vi "UHR-Fleezers Control (host) - Lorentz v3.vi"() -> ()   [LabVIEW 2014] (continued)
            n2217 = property on="APD 2"() -> ("Displayed Image Position"=w3357)  [unwired: 2 in, 2 out]
            n2218 = property on="APD 1"() -> ("Displayed Image Position"=w3386)  [unwired: 2 in, 2 out]
            n2219 = property on="Detection Laser X"() -> ("Displayed Image Position"=w3383)  [unwired: 2 in, 2 out]
            n2220 = property on="Detection Laser Y"() -> ("Displayed Image Position"=w3382)  [unwired: 2 in, 2 out]
            n2221 = Unbundle By Name(w3356) -> ("Width"=w3353, "Height"=w3352)
            n2222 = Unbundle By Name(w3357) -> ("Left"=w3355, "Top"=w3354)
            n2223 = Unbundle By Name(w3384) -> ("Width"=w3378, "Height"=w3377)
            n2224 = Unbundle By Name(w3385) -> ("Width"=w3374, "Height"=w3373)
            n2225 = Unbundle By Name(w3381) -> ("Width"=w3370, "Height"=w3369)
            n2226 = Unbundle By Name(w3386) -> ("Left"=w3380, "Top"=w3379)
            n2227 = Unbundle By Name(w3383) -> ("Left"=w3376, "Top"=w3375)
            n2228 = Unbundle By Name(w3382) -> ("Left"=w3372, "Top"=w3371)
            n2229 = Bundle("Left"=w3355, "Top"=w3354, "Width"=w3353, "Height"=w3352) -> (w3351:T49)  [unwired: 1 in]
            n2230 = Bundle("Left"=w3380, "Top"=w3379, "Width"=w3378, "Height"=w3377) -> (w3368:T49)  [unwired: 1 in]
            n2231 = Bundle("Left"=w3376, "Top"=w3375, "Width"=w3374, "Height"=w3373) -> (w3367:T49)  [unwired: 1 in]
            n2232 = Bundle("Left"=w3372, "Top"=w3371, "Width"=w3370, "Height"=w3369) -> (w3366:T49)  [unwired: 1 in]
            n2233 = Build Cluster Array(w3351, w3368, w3367, w3366) -> (w3365:T50)
            n2234 = for {
              tunnel: w3387 -> [w3398]
              tunnel: w3365 -> [w3399] mode=indexing
              shift-right: [w3396] -> w3363
              shift-left: TRUE -> [w3397]
              shift-right: [w3395] -> w3361
              shift-left: _ -> [w3391]
              shift-right: [w3394] -> w3360
              shift-left: _ -> [w3390]
              shift-right: [w3393] -> w3359
              shift-left: _ -> [w3389]
              shift-right: [w3392] -> w3358
              shift-left: _ -> [w3388]
              n2235 = case shown="True" w3397 {
                selector: w3397 -> [w3404 _]
                tunnel: w3399 -> [_ w3413]
                tunnel: w3398 -> [_ w3411]
                tunnel: [w3404 w3409] -> w3396
                tunnel: [w3403 w3408] -> w3395
                tunnel: [w3402 w3407] -> w3394
                tunnel: [w3401 w3406] -> w3393
                tunnel: [w3400 w3405] -> w3392
                tunnel: w3391 -> [w3403 _]
                tunnel: w3390 -> [w3402 _]
                tunnel: w3389 -> [w3401 _]
                tunnel: w3388 -> [w3400 _]
                frame False {
                }
                frame True {
                  n2236 = Unbundle(w3413) -> (w3412:T49)
                  n2237 = call "isclickinwindow.vi"("Image Param"=w3412, "Point32"=w3411) -> ("4 Y"=w3405:i32, "3 Height"=w3406:i32, "2 X"=w3407:i32, "1 Width"=w3408:i32, "In image?"=w3410:bool)  [unwired: 1 in]
                  n2238 = Not(x=w3410) -> (.not. x?=w3409:bool)
                }
              }
            }
            n2239 = Not(x=w3363) -> (.not. x?=w3362:bool)
            n2240 = case shown="True" w3362 {
              tunnel: w3360 -> [_ w3427]
              tunnel: w3358 -> [_ w3426]
              tunnel: w3361 -> [_ w3425]
              tunnel: w3359 -> [_ w3424]
              frame False {
              }
              frame True {
                w3414 = FALSE ("Get Point")
                n2241 = local read "Scan lines (y)"() -> (w3429:u64)
                n2242 = disable-structure shown="Disabled" {
                  frame Disabled {
                  }
                  frame Enabled {
                  }
                }
                n2243 = local read "Actual MCL Inc (V)"() -> (w3423:dbl)
                n2244 = local read "Scan steps (MCL)"() -> (w3428:u64)
                n2245 = Divide "Y Pix/step"(x=w3424, y=w3429) -> (x/y=w3436:dbl)
                n2246 = Divide "Y V/pix"(x=w3423, y=w3436) -> (x/y=w3435:dbl)
                n2247 = Divide "Y half step offset"(x=w3423, y=2.0) -> (x/y=w3437:dbl)
                n2248 = Divide "X pix/step"(x=w3425, y=w3428) -> (x/y=w3434:dbl)
                n2249 = Negate(x=w3437) -> (-x=w3438:dbl)
                n2250 = local read "Initial Y"() -> (w3444:dbl)
                n2251 = Multiply(x=w3426, y=w3435) -> (x*y=w3445:dbl)
                n2252 = Divide "X half step offset"(x=w3423, y=2.0) -> (x/y=w3431:dbl)
                n2253 = Divide "X V/pix"(x=w3423, y=w3434) -> (x/y=w3433:dbl)
                n2254 = Multiply(x=w3423, y=w3428) -> (x*y=w3440:dbl)
                n2255 = Compound Arithmetic op=ADD(w3438, w3445, w3444) -> (w3415:dbl)
                "Pointer Y (V)" <- w3415
                n2256 = Multiply(x=w3433, y=w3427) -> (x*y=w3442:dbl)
                n2257 = Negate(x=w3431) -> (-x=w3430:dbl)
                n2258 = local read "Initial X"() -> (w3443:dbl)
                n2259 = Negate(x=w3442) -> (-x=w3441:dbl)
                n2260 = Compound Arithmetic op=ADD(w3430, w3440, w3443, w3441) -> (w3416:dbl)
                "Pointer X (V)" <- w3416
                n2261 = case shown="True" "Set High F Confocal Spot (X-Y)" {
                  tunnel: w3416 -> [_ w3446]
                  tunnel: w3415 -> [_ w3447]
                  frame False {
                  }
                  frame True {
                    "Confocal Y 2 (V)" <- w3447
                    "Confocal X 2 (V)" <- w3446
                  }
                }
                n2262 = Or(x="Set X Only", y="Set Confocal Spot (X-Y)") -> (x .or. y?=w3419:bool)
                n2263 = Or(x="Set Confocal Spot (X-Y)", y="Set Y Only") -> (x .or. y?=w3418:bool)
                n2264 = case shown="True" w3419 {
                  tunnel: w3416 -> [_ w3448]
                  frame False {
                  }
                  frame True {
                    n2265 = property on="AO2" class="Slide (strict)"("Val(Sgnl)"=w3448) -> ()  [unwired: 2 in, 2 out]
                    "Confocal X 1 (V)" <- w3448
                  }
                }
                n2266 = case shown="True" w3418 {
                  tunnel: w3415 -> [_ w3449]
                  frame False {
                  }
                  frame True {
                    n2267 = property on="AO1" class="Slide (strict)"("Val(Sgnl)"=w3449) -> ()  [unwired: 2 in, 2 out]
                    "Confocal Y 1 (V)" <- w3449
                  }
                }
                n2268 = local write "Set High F Confocal Spot (X-Y)"(w3414) -> ()
                n2269 = local write "Set Confocal Spot (X-Y)"(w3414) -> ()
                n2270 = local write "Set X Only"(w3414) -> ()
                n2271 = local write "Set Y Only"(w3414) -> ()
              }
            }
          }
          frame 3 {
            n2272 = local read "BD 2 Frequency 1 (MHz)"() -> (w3451:dbl)
            n2273 = local read "BD 1 Frequency 1 (MHz)"() -> (w3452:dbl)
            n2274 = local write "Manipulating Trap"(TRUE ("Manipulating Trap")) -> ()
            n2275 = local write "Coords"(T12 {"Horizontal"=0, "Vertical"=0} ("Coords")) -> ()
            n2276 = while {
              tunnel: w3456 -> [w3461]
              tunnel: w3454 -> [w3460]
              tunnel: w3452 -> [w3459]
              tunnel: w3451 -> [w3458]
              tunnel: w3450 -> [w3457]
              stop <- w3462 stop-if-true
              n2277 = event shown="[0] \"Pane\": Mouse Move" {
                selector: _ -> [_ _]
                dyn-events: _ -> [_ _]
                timeout: _ -> [_ _]
                tunnel: ["Force Manip Abort" w3526] -> w3462
                tunnel: w3461 -> [w3469 _]
                tunnel: w3460 -> [w3467 _]
                tunnel: w3459 -> [w3466 _]
                tunnel: w3458 -> [w3465 _]
                tunnel: w3457 -> [w3463 _]
                event Mouse Move {
                  n2278 = event-data() -> ("Time"=w3470:u32, "Coords"=w3471:T12)  [unwired: 3 out]
                  n2279 = Less?(x=w3470, y=w3469) -> (x < y?=w3468:bool)
                  n2280 = case "Makes sure old motion events prior to mouse click aren't used" shown="False" w3468 {
                    tunnel: w3471 -> [w3513 _]
                    tunnel: w3467 -> [w3514 _]
                    tunnel: w3466 -> [w3488 _]
                    tunnel: w3465 -> [w3487 _]
                    tunnel: w3463 -> [w3472 _]
                    frame False {
                      n2281 = Subtract(x=w3513, y=w3514) -> (x-y=w3512:T12)
                      "Coords" <- w3512
                      n2282 = local read "Y RF Frequency Limits (MHz)"() -> (w3473:T24)
                      n2283 = To Double Precision Float(number=w3512) -> (double precision float=w3511:cluster{"Horizontal":dbl, "Vertical":dbl})
                      n2284 = Multiply(x=cluster{"Horizontal":dbl, "Vertical":dbl} {"Horizontal"=-1.0, "Vertical"=1.0}, y="Manipulation Scaling") -> (x*y=w3507:cluster{"Horizontal":dbl, "Vertical":dbl})
                      n2285 = local read "X RF Frequency Limits (MHz)"() -> (w3474:T24)
                      n2286 = Multiply(x=w3511, y=w3507) -> (x*y=w3509:cluster{"Horizontal":dbl, "Vertical":dbl})
                      n2287 = Unbundle By Name(w3509) -> ("Horizontal"=w3504:dbl, "Vertical"=w3508:dbl)
                      n2288 = Unbundle By Name(w3473) -> ("Maximum"=w3476:dbl, "Minimum"=w3475:dbl)
                      n2289 = Boolean To (0,1)(Boolean="Manip. X?") -> (0, 1=w3502:i16)
                      n2290 = Boolean To (0,1)(Boolean="Manip. Y?") -> (0, 1=w3499:i16)
                      n2291 = local read "BD 1 Frequency 2 (MHz)"() -> (w3490:dbl)
                      n2292 = Multiply(x=w3508, y=w3499) -> (x*y=w3501:dbl)
                      n2293 = Multiply(x=w3502, y=w3504) -> (x*y=w3505:dbl)
                      n2294 = local read "BD 2 Frequency 2 (MHz)"() -> (w3489:dbl)
                      n2295 = Unbundle By Name(w3474) -> ("Maximum"=w3478:dbl, "Minimum"=w3477:dbl)
                      n2296 = Add(x=w3487, y=w3501) -> (x+y=w3480:dbl)
                      n2297 = Add(x=w3488, y=w3505) -> (x+y=w3482:dbl)
                      n2298 = In Range and Coerce(upper limit=w3478, x=w3482, lower limit=w3477) -> (coerced(x)=w3481:dbl)  [unwired: 1 out]
                      n2299 = In Range and Coerce(upper limit=w3476, x=w3480, lower limit=w3475) -> (coerced(x)=w3479:dbl)  [unwired: 1 out]
                      n2300 = Subtract(x=w3481, y=w3490) -> (x-y=w3498:dbl)
                      n2301 = Subtract(x=w3479, y=w3489) -> (x-y=w3497:dbl)
                      n2302 = Square(x=w3498) -> (x^2=w3496:dbl)
                      n2303 = Square(x=w3497) -> (x^2=w3495:dbl)
                      n2304 = Add(x=w3496, y=w3495) -> (x+y=w3494:dbl)
                      n2305 = Square Root(x=w3494) -> (sqrt(x)=w3491:dbl)
                      n2306 = In Range and Coerce(upper limit="Limit Max (MHz)", x=w3491, lower limit="Limit Min (MHz)") -> (In Range?=w3484:bool)  [unwired: 1 out]
                      n2307 = Not(x="Limits Enable") -> (.not. x?=w3483:bool)
                      n2308 = Or(x=w3484, y=w3483) -> (x .or. y?=w3485:bool)
                      n2309 = case shown="True" w3485 {
                        tunnel: w3491 -> [_ w3516]
                        tunnel: w3481 -> [_ w3523]
                        tunnel: w3490 -> [_ w3522]
                        tunnel: w3479 -> [_ w3521]
                        tunnel: w3489 -> [_ w3520]
                        tunnel: w3474 -> [_ w3518]
                        tunnel: w3473 -> [_ w3517]
                        tunnel: w3472 -> [_ w3515]
                        frame False {
                        }
                        frame True {
                          n2310 = local read "BD 1 Frequency 3 (MHz)"() -> (w3524:dbl)
                          n2311 = local read "BD 2 Frequency 3 (MHz)"() -> (w3519:dbl)
                          n2312 = local write "Trap Delta (MHz)"(w3516) -> ()
                          n2313 = call "set RF board frequency - interlace.vi"("Board 2 Frequency Limits"=w3517, "Board 1 Frequency Limits"=w3518, "FPGA VI Reference In"=w3515, "Board 2 Frequency 3 (MHz)"=w3519, "Board 1 Frequency 3 (MHz)"=w3524, "Board 2 Frequency 2 (MHz)"=w3520, "Board 2 Frequency 1 (MHz)"=w3521, "Board 1 Frequency 2 (MHz)"=w3522, "Board 1 Frequency 1  (MHz)"=w3523) -> ()  [unwired: 1 in, 2 out]
                          n2314 = local write "BD 2 Frequency 1 (MHz)"(w3521) -> ()
                          n2315 = local write "BD 1 Frequency 1 (MHz)"(w3523) -> ()
                        }
                      }
                    }
                    frame True {
                    }
                  }
                }
                event Mouse Up {
                  n2316 = event-data() -> ("Button"=w3525:u16)  [unwired: 8 out]
                  n2317 = case shown="3" w3525 {
                    tunnel: [FALSE TRUE] -> w3526
                    frame 0, Default {
                    }
                    frame 3 {
                      n2318 = local read "Trap Delta (MHz)"() -> (w3528:dbl)
                      n2319 = property on="Initial delta (MHz)" class="DigNum (strict)"("Val(Sgnl)"=w3528) -> ()  [unwired: 2 in, 2 out]
                      n2320 = local write "Manipulating Trap"(FALSE ("Manipulating Trap")) -> ()
                    }
                  }
                }
              }
            }
          }
        }
      }
      event Timeout {
        n2321 = event-data() -> ()  [unwired: 4 out]
      }
      event "Stop All": Mouse Down {
        n2322 = event-data() -> ()  [unwired: 9 out]
      }
      event Mouse Move {
        n2323 = event-data() -> ()  [unwired: 6 out]
      }
    }
    n2324 = node-c288() -> ()  [unwired: 2 out]
  }
  n2325 = node-c288(3 ("Processor")) -> (w63:T37)  [unwired: 3 out]
  n2326 = node-c288(i64 1 ("Period"), 1 ("Processor")) -> (w71:T37)  [unwired: 2 in, 2 out]
  n2327 = timed-loop "Oscillate Trap/AOM (fishing, conjugate plane alignment)" {
    tunnel: [w3534] -> w68
    timing: w63 -> [_]
    timing-out: [_] -> w62
    tunnel: w24 -> [w3533]
    tunnel: w12 -> [w3532]
    stop <- w3534 stop-if-true
    n2328 = node-c288() -> ()  [unwired: 2 out]
    n2329 = event shown="[2] \"Start assembly line\": Value Change" {
      selector: _ -> [_ _ _ _]
      dyn-events: _ -> [_ _ _ _]
      timeout: _ -> [_ _ _ _]
      tunnel: [FALSE ("Stop All") _ _ w4207] -> w3534
      tunnel: w3533 -> [w3537 _ _ _]
      tunnel: w3532 -> [_ _ w4142 _]
      event "Oscillate Set 1", "Fish for Tether": Value Change {
        n2330 = event-data() -> ()  [unwired: 6 out]
        n2331 = local read "Oscillate Set 1"() -> (w3541:bool)
        n2332 = Or(x=w3541, y="Fish for Tether") -> (x .or. y?=w3539:bool)
        n2333 = case shown="True" w3539 {
          tunnel: "Fish for Tether" -> [_ w3544]
          tunnel: w3537 -> [_ w3542]
          frame False {
          }
          frame True {
            n2334 = case shown="True" w3544 {
              selector: w3544 -> [w3547 w3553]
              tunnel: [w3547 w3553] -> w3543
              frame False {
              }
              frame True {
                n2335 = local write "Scan axis 2"(TRUE) -> ()
                n2336 = local write "Tether"(FALSE ("Tether")) -> ()
                n2337 = local read "Flow ON during cal?"() -> (w3548:bool)
                n2338 = property on="Trap Delta (MHz)" class="DigNum (strict)"("Val(Sgnl)"="Furthest Delta (MHz)") -> ()  [unwired: 2 in, 2 out]
                n2339 = Or(x="Flow ON during \nfishing?", y=w3548) -> (x .or. y?=w3549:bool)
                n2340 = Wait (ms)(milliseconds to wait=u32 500) -> ()  [unwired: 1 out]
                n2341 = property on="Sample Channel\nFlow" class="Bool (strict)"("Val(Sgnl)"=w3549) -> ()  [unwired: 2 in, 2 out]
              }
            }
            n2342 = node-c288() -> (w3546:T37)  [unwired: 1 in, 3 out]
            n2343 = timed-loop "Oscillate AOD" {
              timing: w3546 -> [_]
              timing-out: [_] -> w3545
              tunnel: w3543 -> [w3557]
              tunnel: w3542 -> [w3556]
              i -> [w3565]
              stop <- w3563 stop-if-true
              n2344 = node-c288() -> (w3564:i64)  [unwired: 1 out]
              n2345 = flat-sequence {
                tunnel: w3565 -> [w3592]
                tunnel: w3564 -> [w3591]
                tunnel: w3557 -> [w3575]
                tunnel: [w3575] -> w3562
                tunnel: [w3574] -> w3561
                tunnel: [w3573] -> w3560
                tunnel: [w3570] -> w3558
                tunnel: w3556 -> [w3566]
                tunnel: w3562 -> [w3639]
                tunnel: w3561 -> [w3637]
                tunnel: w3560 -> [w3636]
                tunnel: [w3635] -> w3559
                tunnel: w3558 -> [w3634]
                tunnel: [w3711] -> w3563
                tunnel: w3559 -> [w3710]
                frame #0 {
                  # "w (rad/s)"
                  # "t (s)"
                  n2346 = Divide(x=w3591, y=i64 1000) -> (x/y=w3567:dbl)
                  n2347 = local read "BD 1 Frequency 2 (MHz)"() -> (w3569:dbl)
                  n2348 = Multiply(x="Osc. freq. (Hz)", y=6.283185307179586) -> (x*y=w3589:dbl)
                  n2349 = Multiply(x=w3567, y=w3592) -> (x*y=w3588:dbl)
                  n2350 = Multiply(x=w3589, y=w3588) -> (x*y=w3572:dbl)
                  n2351 = local read "BD 1 Frequency 1 (MHz)"() -> (w3577:dbl)
                  n2352 = case shown="True" w3575 {
                    tunnel: w3572 -> [w3598 w3617]
                    tunnel: w3577 -> [_ w3625]
                    tunnel: w3569 -> [_ w3626]
                    tunnel: [w3595 w3621] -> w3568
                    tunnel: [FALSE w3599] -> w3573
                    tunnel: [0.0 w3613] -> w3570
                    frame False {
                      n2353 = Sine(x=w3598) -> (sin(x)=w3596:dbl)
                      n2354 = Multiply(x=w3596, y="Osc. amp. (MHz)") -> (x*y=w3595:dbl)
                    }
                    frame True {
                      # "trap position goes from 0 to 1 (0 is when it is furthest away, 1 is when closest)\nso we want to test for tether only when farther away, or x < 1"
                      # "quit if taking too long"
                      # "oscillate the trap"
                      # "Test for tether"
                      n2355 = local read "Vec Mean of T1 T2"() -> (w3602:dbl[])
                      "Trigger Signal" <- w3602
                      n2356 = Cosine(x=w3617) -> (cos(x)=w3629:dbl)
                      n2357 = Subtract(x=w3626, y=w3625) -> (x-y=w3624:dbl)
                      n2358 = Decrement(x=w3629) -> (x-1=w3628:dbl)
                      n2359 = Subtract(x=w3624, y="Closest Delta (MHz)") -> (x-y=w3622:dbl)
                      n2360 = Divide(x=w3628, y=-2.0) -> (x/y=w3612:dbl)
                      n2361 = Greater?(x=w3602, y="Stop F (pN)") -> (0:w3619:bool[])
                      n2362 = Multiply(x=w3612, y=w3622) -> (x*y=w3621:dbl)
                      n2363 = Less?(x=w3612, y="Fish mask thresh") -> (x < y?=w3611:bool)
                      n2364 = Boolean To (0,1)(Boolean=w3611) -> (0, 1=w3609:i16)
                      n2365 = Multiply(x=w3609, y=w3602) -> (x*y=w3608:dbl[])
                      n2366 = Divide(x=w3617, y=6.283185307179586) -> (x/y=w3616:dbl)
                      n2367 = Round Toward +Infinity(x=w3616) -> (ceil(x): smallest int >= x=w3613:dbl)
                      "Attempts" <- w3613
                      n2368 = Greater?(x=w3608, y="Stop F (pN) (mask)") -> (0:w3606:bool[])
                      n2369 = Or Array Elements(Boolean array=w3619) -> (logical OR=w3604:bool)
                      n2370 = Or Array Elements(Boolean array=w3606) -> (logical OR=w3603:bool)
                      n2371 = Greater?(x=w3613, y="Attempt Limit") -> (0:w3615:bool)
                      n2372 = case shown="True" w3615 {
                        frame False {
                        }
                        frame True {
                          n2373 = local write "Fish for Tether"(FALSE ("Fish for Tether")) -> ()
                          n2374 = call <vilib>:"Beep.vi"() -> ()  [unwired: 3 in, 9 out]
                          n2375 = local read "Messages"() -> (w3631:string)
                          n2376 = call "Update messages.vi"("Message to add"="Tether fishing timeout." ("Messages"), "Old message string"=w3631) -> ("New message string"=→"Messages":string)
                        }
                      }
                      n2377 = Select(t=w3604, s="Normal (on) or masked test (off)", f=w3603) -> (s? t:f=w3601:bool)
                      n2378 = And(x="Stop Fishing When Tether", y=w3601) -> (x .and. y?=w3599:bool)
                    }
                  }
                  n2379 = local read "BD 2 Frequency 1 (MHz)"() -> (w3576:dbl)
                  n2380 = Select(t=w3577, s="Scan axis 2", f=w3576) -> (s? t:f=w3580:dbl)
                  n2381 = Add(x=w3568, y=w3580) -> (x+y=w3574:dbl)
                  n2382 = Select(t=w3574, s="Scan axis 2", f=w3577) -> (s? t:f=w3583:dbl)
                  n2383 = Select(t=w3576, s="Scan axis 2", f=w3574) -> (s? t:f=w3582:dbl)
                  n2384 = local read "BD 2 Frequency 2 (MHz)"() -> (w3585:dbl)
                  n2385 = local read "BD 2 Frequency 3 (MHz)"() -> (w3584:dbl)
                  n2386 = local read "Y RF Frequency Limits (MHz)"() -> (w3578:T24)
                  n2387 = local read "X RF Frequency Limits (MHz)"() -> (w3579:T24)
                  n2388 = local read "BD 1 Frequency 3 (MHz)"() -> (w3586:dbl)
                  n2389 = call "set RF board frequency - interlace.vi"("Board 2 Frequency Limits"=w3578, "Board 1 Frequency Limits"=w3579, "FPGA VI Reference In"=w3566, "Board 2 Frequency 3 (MHz)"=w3584, "Board 1 Frequency 3 (MHz)"=w3586, "Board 2 Frequency 2 (MHz)"=w3585, "Board 2 Frequency 1 (MHz)"=w3582, "Board 1 Frequency 2 (MHz)"=w3569, "Board 1 Frequency 1  (MHz)"=w3583) -> ()  [unwired: 1 in, 2 out]
                }
                frame #1 {
                  n2390 = And(x=w3639, y=w3636) -> (x .and. y?=w3638:bool)
                  n2391 = case "Only if were fishing and now formed tether" shown="True" w3638 {
                    tunnel: w3637 -> [w3641 w3656]
                    tunnel: [w3640 w3655] -> w3635
                    tunnel: w3634 -> [_ w3651]
                    frame False {
                      n2392 = local read "Fish for Tether"() -> (w3640:bool)
                      n2393 = case shown="False" w3640 {
                        tunnel: w3641 -> [w3642 _]
                        frame False {
                          n2394 = property on="BD 1 Frequency 1 (MHz)" class="DigNum (strict)"("Val(Sgnl)"=w3642) -> ()  [unwired: 2 in, 2 out]
                        }
                        frame True {
                        }
                      }
                    }
                    frame True {
                      w3655 = FALSE ("Fish for Tether")
                      n2395 = call <vilib>:"Beep.vi"() -> ()  [unwired: 3 in, 9 out]
                      n2396 = Number To Decimal String(number=w3651, width (-)=i16 1) -> (decimal integer string=w3649:string)
                      n2397 = Concatenate Strings("Formed tether in ", w3649, " attempt(s)." ("string")) -> (w3646:string)
                      n2398 = local read "Messages"() -> (w3653:string)
                      n2399 = local write "Fish for Tether"(w3655) -> ()
                      n2400 = call "Update messages.vi"("Message to add"=w3646, "Old message string"=w3653) -> ("New message string"=w3652:string)
                      n2401 = local write "Messages"(w3652) -> ()
                      n2402 = Get Date/Time In Seconds() -> (seconds since 1Jan1904=→"Time tether formed":timestamp)
                      n2403 = local read "Flow ON during cal?"() -> (w3643:bool)
                      n2404 = property on="Sample Channel\nFlow" class="Bool (strict)"("Val(Sgnl)"=w3643) -> (error out=w3644:errorcluster)  [unwired: 2 in, 1 out]
                      n2405 = case shown="\"2\", \"3\", \"4\", \"5\", \"6\"" "Then..." {
                        selector: "Then..." -> [_ w3659]
                        tunnel: w3656 -> [w3658 _]
                        tunnel: w3644 -> [_ _]
                        frame "1", Default {
                          n2406 = property on="BD 1 Frequency 1 (MHz)" class="DigNum (strict)"("Val(Sgnl)"=w3658) -> ()  [unwired: 2 in, 2 out]
                        }
                        frame "2", "3", "4", "5", "6" {
                          n2407 = flat-sequence {
                            tunnel: w3659 -> [w3661]
                            frame #0 {
                              n2408 = property on="Trap Delta (MHz)" class="DigNum (strict)"("Val(Sgnl)"="Move to Delta 1 (MHz)") -> ()  [unwired: 2 in, 2 out]
                            }
                            frame #1 {
                              n2409 = case shown="\"5\", \"6\"" w3661 {
                                selector: w3661 -> [w3664 w3674 _]
                                frame "3", "4" {
                                n2410 = flat-sequence {
                                tunnel: w3664 -> [w3665]
                                tunnel: [w3665] -> w3662
                                tunnel: [w3667] -> w3663
                                tunnel: w3662 -> [w3667]
                                tunnel: w3663 -> [w3671]
                                frame #0 {
                                n2411 = property on="Green Laser ON" class="Bool (strict)"("Val(Sgnl)"=TRUE ("Value (Signaling)")) -> ()  [unwired: 2 in, 2 out]
                                }
                                frame #1 {
                                n2412 = Multiply(x="Wait Before Save (s)", y=u32 1000 ("x")) -> (x*y=w3669:u32)
                                n2413 = Wait (ms)(milliseconds to wait=w3669) -> ()  [unwired: 1 out]
                                }
                                frame #2 {
                                n2414 = property on="Start Saving" class="Bool (strict)"("Value"=TRUE ("Start Saving")) -> ()  [unwired: 2 in, 2 out]
                                n2415 = case shown="\"4\"" w3671 {
                                frame Default {
                                }
                                frame "4" {
                                n2416 = property on="Fl. Triggered..." class="Bool (strict)"("Val(Sgnl)"=TRUE ("Value (Signaling)")) -> ()  [unwired: 2 in, 2 out]
                                }
                                }
                                }
                                }
                                }
                                frame "5", "6" {
                                n2417 = stacked-sequence {
                                tunnel: w3674 -> [_ _ _ _ _ _ w3686]
                                frame #0 {
                                n2418 = Replace Array Subset(array=u32[] [0] ("Index Values"), new element="Raster Set Upon Tether", index=0) -> (w3675:u32[])
                                n2419 = property on="Saved AOD Raster Scan Parameter Sets" class="Arr (strict)"("Index Values"=w3675) -> ()  [unwired: 2 in, 2 out]
                                }
                                frame #1 {
                                n2420 = Wait (ms)(milliseconds to wait=u32 500) -> ()  [unwired: 1 out]
                                }
                                frame #2 {
                                n2421 = property on="Load parameters" class="Bool (strict)"("Val(Sgnl)"=TRUE ("Value (Signaling)")) -> ()  [unwired: 2 in, 2 out]
                                n2422 = case shown="True" "Green ON During Raster" {
                                frame False {
                                }
                                frame True {
                                n2423 = property on="Green Laser ON" class="Bool (strict)"("Val(Sgnl)"=TRUE ("Value (Signaling)")) -> ()  [unwired: 2 in, 2 out]
                                }
                                }
                                }
                                frame #3 {
                                n2424 = Wait (ms)(milliseconds to wait=u32 500) -> ()  [unwired: 1 out]
                                }
                                frame #4 {
                                n2425 = property on="Trap Raster Scan" class="Bool (strict)"("Val(Sgnl)"=TRUE ("Value (Signaling)")) -> ()  [unwired: 2 in, 2 out]
                                }
                                frame #5 {
                                n2426 = Wait (ms)(milliseconds to wait=u32 2000) -> ()  [unwired: 1 out]
                                }
                                frame #6 {
                                n2427 = flat-sequence {
                                tunnel: w3686 -> [w3693]
                                frame #0 {
                                n2428 = while {
                                stop <- w3689 stop-if-true
                                n2429 = local read "Raster Scanning..."() -> (w3688:bool)
                                n2430 = local read "Saving..."() -> (w3691:bool)
                                n2431 = Wait (ms)(milliseconds to wait=u32 100) -> ()  [unwired: 1 out]
                                n2432 = Not(x=w3691) -> (.not. x?=w3690:bool)
                                n2433 = Not(x=w3688) -> (.not. x?=w3687:bool)
                                n2434 = And(x=w3690, y=w3687) -> (x .and. y?=w3689:bool)
                                }
                                }
                                frame #1 {
                                n2435 = local read "Tether"() -> (w3694:bool)
                                n2436 = case shown="True" w3694 {
                                tunnel: w3693 -> [_ w3696]
                                frame False {
                                n2437 = property on="Fish for Tether" class="Bool (strict)"("Val(Sgnl)"="Fish again after \nraster break?") -> ()  [unwired: 2 in, 2 out]
                                }
                                frame True {
                                n2438 = stacked-sequence {
                                tunnel: w3696 -> [_ w3700 _ _]
                                frame #0 {
                                n2439 = property on="Trap Delta (MHz)" class="DigNum (strict)"("Val(Sgnl)"="Move to Delta 2 (MHz)") -> ()  [unwired: 2 in, 2 out]
                                n2440 = case shown="True" "Flow ON after\ntether testing?" {
                                frame False {
                                }
                                frame True {
                                n2441 = property on="Sample Channel\nFlow" class="Bool (strict)"("Val(Sgnl)"=TRUE ("Value (Signaling)")) -> ()  [unwired: 2 in, 2 out]
                                }
                                }
                                }
                                frame #1 {
                                n2442 = flat-sequence {
                                tunnel: w3700 -> [w3702]
                                frame #0 {
                                n2443 = Wait (ms)(milliseconds to wait=u32 500) -> ()  [unwired: 1 out]
                                }
                                frame #1 {
                                n2444 = case shown="\"6\"" w3702 {
                                frame Default {
                                }
                                frame "6" {
                                n2445 = property on="Green Laser ON" class="Bool (strict)"("Val(Sgnl)"=TRUE ("Green Laser ON/Interlacing")) -> ()  [unwired: 2 in, 2 out]
                                }
                                }
                                }
                                frame #2 {
                                n2446 = Wait (ms)(milliseconds to wait=u32 500) -> ()  [unwired: 1 out]
                                }
                                frame #3 {
                                n2447 = local write "Start Saving"("Save at end (5, 6)") -> ()
                                }
                                }
                                }
                                frame #2 {
                                n2448 = local read "Bead Sep. Int. Time (s)"() -> (w3708:dbl)
                                n2449 = Multiply(x=w3708, y=1000.0) -> (x*y=w3707:dbl)
                                n2450 = Wait (ms)(milliseconds to wait=w3707) -> ()  [unwired: 1 out]
                                }
                                frame #3 {
                                n2451 = property on="Remove Offset" class="Bool (strict)"("Val(Sgnl)"=TRUE ("Value (Signaling)")) -> ()  [unwired: 2 in, 2 out]
                                }
                                }
                                }
                                }
                                }
                                }
                                }
                                }
                                }
                                frame "2", Default {
                                }
                              }
                            }
                          }
                        }
                      }
                      "Tether" <- "Tether Alarm?"
                    }
                  }
                }
                frame #2 {
                  n2452 = local read "Oscillate Set 1"() -> (w3715:bool)
                  n2453 = local read "Stop All"() -> (w3713:bool)
                  n2454 = Or(x=w3715, y=w3710) -> (x .or. y?=w3712:bool)
                  n2455 = Not(x=w3712) -> (.not. x?=w3714:bool)
                  n2456 = Compound Arithmetic op=OR(w3713, w3714) -> (w3711:bool)
                }
              }
              n2457 = node-c288() -> ()  [unwired: 2 out]
            }
            n2458 = node-c288(w3545) -> ()  [unwired: 1 out]
          }
        }
      }
      event "Fl. Triggered...": Value Change {
        n2459 = event-data() -> ()  [unwired: 7 out]
        n2460 = case shown="True" "Fl. Triggered..." {
          frame False {
          }
          frame True {
            n2461 = node-c288() -> (w3726:T37)  [unwired: 4 out]
            n2462 = timed-loop {
              timing: w3726 -> [_]
              timing-out: [_] -> w3725
              tunnel: "Action" -> [w3734]
              shift-right: [w3731] -> _
              shift-left: u8 255 -> [w3733]
              shift-right: [w3728] -> _
              shift-left: 255 -> [w3730]
              stop <- w3727 stop-if-true
              # "Reset confocal spot"
              n2463 = node-c288() -> ()  [unwired: 2 out]
              n2464 = flat-sequence {
                tunnel: w3734 -> [w3754]
                tunnel: w3733 -> [w3753]
                tunnel: [w3752] -> w3732
                tunnel: w3730 -> [w3739]
                tunnel: [w3738] -> w3729
                tunnel: [w4133] -> w3727
                tunnel: w3732 -> [w4132]
                tunnel: [w4132] -> w3731
                tunnel: [w4131] -> w3728
                tunnel: w3729 -> [w4131]
                frame #0 {
                  n2465 = local read "Delta Fl. 2"() -> (w3751:dbl)
                  n2466 = local read "Delta Fl. 1"() -> (w3746:dbl)
                  n2467 = Multiply(x="Fl. Delta Thresh. (kHz)", y=1000.0) -> (x*y=w3741:dbl)
                  n2468 = Select(t=w3746, s="APD to Watch", f=w3751) -> (s? t:f=w3742:dbl)
                  n2469 = Greater?(x=w3742, y=w3741) -> (0:w3747:bool)
                  n2470 = Or(x="Force Yank", y=w3747) -> (x .or. y?=w3745:bool)
                  n2471 = And(x=w3745, y="Yank when?") -> (x .and. y?=w3743:bool)
                  n2472 = case shown="True" w3743 {
                    tunnel: w3754 -> [w3757 w3958]
                    tunnel: w3753 -> [w3759 w3954]
                    tunnel: [w3759 w3952] -> w3752
                    tunnel: w3742 -> [w3765 _]
                    tunnel: w3741 -> [w3764 _]
                    tunnel: "Force Yank" -> [w3762 _]
                    tunnel: w3739 -> [w3761 w3951]
                    tunnel: [w3760 w3951] -> w3738
                    frame False {
                      n2473 = Negate(x=w3764) -> (-x=w3756:dbl)
                      n2474 = local write "Fl. High"(TRUE ("Fl. High")) -> ()
                      n2475 = Less?(x=w3765, y=w3756) -> (x < y?=w3763:bool)
                      n2476 = Or(x=w3762, y=w3763) -> (x .or. y?=w3758:bool)
                      n2477 = case shown="True" w3758 {
                        tunnel: w3761 -> [w3766 w3776]
                        tunnel: [w3766 w3775] -> w3760
                        tunnel: w3757 -> [_ w3774]
                        frame False {
                        }
                        frame True {
                          n2478 = flat-sequence {
                            tunnel: w3776 -> [w3782]
                            tunnel: w3774 -> [w3779]
                            tunnel: [w3781] -> w3773
                            tunnel: [w3780] -> w3772
                            tunnel: [w3779] -> w3771
                            tunnel: w3770 -> [w3778]
                            tunnel: [w3778] -> w3769
                            tunnel: w3768 -> [w3777]
                            tunnel: [w3777] -> w3767
                            tunnel: [w3853] -> w3775
                            tunnel: w3773 -> [w3853]
                            tunnel: w3772 -> [w3852]
                            tunnel: w3771 -> [w3851]
                            tunnel: w3769 -> [w3850]
                            tunnel: w3767 -> [w3849]
                            frame #0 {
                              n2479 = call <vilib>:"Beep.vi"() -> ()  [unwired: 12 in]
                              n2480 = local write "Waiting"(FALSE ("Waiting")) -> ()
                              n2481 = Increment(x=w3782) -> (x+1=w3781:i32)
                              n2482 = case shown="\"Image\"" w3779 {
                                tunnel: w3781 -> [_ w3787 _]
                                frame "Alarm", Default {
                                }
                                frame "Yank" {
                                n2483 = flat-sequence {
                                tunnel: w3787 -> [w3790]
                                tunnel: [w3789] -> w3786
                                tunnel: [w3788] -> w3785
                                tunnel: w3786 -> [w3800]
                                tunnel: w3785 -> [w3801]
                                frame #0 {
                                n2484 = local read "Yank Delay (s)"() -> (w3793:dbl)
                                n2485 = local read "N Array El"() -> (w3788:u8)
                                n2486 = Quotient & Remainder(x=w3790, y=w3788) -> (x-y*floor(x/y)=w3789:i32)  [unwired: 1 out]
                                n2487 = Multiply(x=w3793, y=1000.0) -> (x*y=w3791:dbl)
                                n2488 = Wait (ms)(milliseconds to wait=w3791) -> ()  [unwired: 1 out]
                                }
                                frame #1 {
                                n2489 = local read "Yank to which?"() -> (w3795:bool)
                                n2490 = local read "Random Choice"() -> (w3805:bool)
                                n2491 = local read "Yank to Trap Delta (MHz)"() -> (w3798:dbl[])
                                n2492 = local read "Yank to SP"() -> (w3799:dbl[])
                                n2493 = Random Number (0-1)() -> (number: 0 to 1=w3804:dbl)
                                n2494 = Multiply(x=w3801, y=w3804) -> (x*y=w3803:dbl)
                                n2495 = Round Toward -Infinity(1:w3803) -> (0:w3802:dbl)
                                n2496 = Select(t=w3802, s=w3805, f=w3800) -> (s? t:f=w3796:dbl)
                                n2497 = Select(t=w3798, s=w3795, f=w3799) -> (s? t:f=w3797:dbl[])
                                n2498 = Index Array(array=w3797, index=w3796) -> (element=w3794:dbl)
                                n2499 = case shown="True" w3795 {
                                tunnel: w3794 -> [w3806 w3833]
                                frame False {
                                n2500 = flat-sequence {
                                tunnel: w3806 -> [w3807]
                                frame #0 {
                                n2501 = property on="Trap Pos FB SP" class="DigNum (strict)"("Val(Sgnl)"=w3807) -> ()  [unwired: 2 in, 2 out]
                                }
                                frame #1 {
                                n2502 = Wait (ms)(milliseconds to wait=u32 700) -> ()  [unwired: 1 out]
                                }
                                frame #2 {
                                n2503 = local read "Action (%)"() -> (w3812:dbl)
                                n2504 = Absolute Value(x=w3812) -> (abs(x)=w3811:dbl)
                                n2505 = Greater?(x=w3811, y=70.0) -> (0:w3809:bool)
                                n2506 = property on="Remove Action Offset" class="Bool (strict)"("Val(Sgnl)"=w3809) -> ()  [unwired: 2 in, 2 out]
                                }
                                frame #3 {
                                n2507 = for {
                                N: 4 -> [_]
                                n2508 = flat-sequence {
                                frame #0 {
                                n2509 = Wait (ms)(milliseconds to wait=u32 500) -> ()  [unwired: 1 out]
                                }
                                frame #1 {
                                n2510 = local read "Action (%)"() -> (w3818:dbl)
                                n2511 = Absolute Value(x=w3818) -> (abs(x)=w3817:dbl)
                                n2512 = Greater?(x=w3817, y=70.0) -> (0:w3815:bool)
                                n2513 = property on="Remove Action Offset" class="Bool (strict)"("Val(Sgnl)"=w3815) -> ()  [unwired: 2 in, 2 out]
                                }
                                }
                                }
                                }
                                frame #4 {
                                n2514 = Wait (ms)(milliseconds to wait=u32 500) -> ()  [unwired: 1 out]
                                }
                                frame #5 {
                                n2515 = local read "Mean"() -> (w3826:dbl)
                                n2516 = Greater?(x=w3826, y=11.0) -> (0:w3820:bool)
                                n2517 = Not(x=w3820) -> (.not. x?=w3821:bool)
                                n2518 = And(x=w3821, y="Shift confocal") -> (x .and. y?=w3823:bool)
                                n2519 = And(x=w3820, y="Shift confocal") -> (x .and. y?=w3824:bool)
                                n2520 = case shown="True" w3824 {
                                frame False {
                                }
                                frame True {
                                n2521 = local read "Confocal Y 2 (V)"() -> (w3830:dbl)
                                n2522 = local read "Confocal X 2 (V)"() -> (w3829:dbl)
                                n2523 = property on="AO1" class="Slide (strict)"("Val(Sgnl)"=w3830) -> ()  [unwired: 2 in, 2 out]
                                n2524 = property on="AO2" class="Slide (strict)"("Val(Sgnl)"=w3829) -> ()  [unwired: 2 in, 2 out]
                                }
                                }
                                n2525 = case shown="True" w3823 {
                                frame False {
                                }
                                frame True {
                                n2526 = local read "Confocal Y 1 (V)"() -> (w3828:dbl)
                                n2527 = local read "Confocal X 1 (V)"() -> (w3827:dbl)
                                n2528 = property on="AO1" class="Slide (strict)"("Val(Sgnl)"=w3828) -> ()  [unwired: 2 in, 2 out]
                                n2529 = property on="AO2" class="Slide (strict)"("Val(Sgnl)"=w3827) -> ()  [unwired: 2 in, 2 out]
                                }
                                }
                                }
                                frame #6 {
                                n2530 = Wait (ms)(milliseconds to wait=u32 1500) -> ()  [unwired: 1 out]
                                }
                                frame #7 {
                                n2531 = property on="Rem fb disp offset" class="Bool (strict)"("Val(Sgnl)"=TRUE ("Value (Signaling)")) -> ()  [unwired: 2 in, 2 out]
                                }
                                }
                                }
                                frame True {
                                n2532 = flat-sequence {
                                tunnel: w3833 -> [w3834]
                                frame #0 {
                                n2533 = property on="Trap Delta (MHz)" class="DigNum (strict)"("Val(Sgnl)"=w3834) -> ()  [unwired: 2 in, 2 out]
                                }
                                frame #1 {
                                n2534 = Wait (ms)(milliseconds to wait=u32 500) -> ()  [unwired: 1 out]
                                }
                                frame #2 {
                                n2535 = local read "Shift confocal"() -> (w3840:bool)
                                n2536 = local read "Mean"() -> (w3842:dbl)
                                n2537 = Greater?(x=w3842, y=11.0) -> (0:w3839:bool)
                                n2538 = Not(x=w3839) -> (.not. x?=w3838:bool)
                                n2539 = And(x=w3838, y=w3840) -> (x .and. y?=w3836:bool)
                                n2540 = And(x=w3839, y=w3840) -> (x .and. y?=w3837:bool)
                                n2541 = case shown="True" w3837 {
                                frame False {
                                }
                                frame True {
                                n2542 = local read "Confocal Y 2 (V)"() -> (w3846:dbl)
                                n2543 = local read "Confocal X 2 (V)"() -> (w3845:dbl)
                                n2544 = property on="AO2" class="Slide (strict)"("Val(Sgnl)"=w3845) -> ()  [unwired: 2 in, 2 out]
                                n2545 = property on="AO1" class="Slide (strict)"("Val(Sgnl)"=w3846) -> ()  [unwired: 2 in, 2 out]
                                }
                                }
                                n2546 = case shown="True" w3836 {
                                frame False {
                                }
                                frame True {
                                n2547 = local read "Confocal X 1 (V)"() -> (w3843:dbl)
                                n2548 = local read "Confocal Y 1 (V)"() -> (w3844:dbl)
                                n2549 = property on="AO2" class="Slide (strict)"("Val(Sgnl)"=w3843) -> ()  [unwired: 2 in, 2 out]
                                n2550 = property on="AO1" class="Slide (strict)"("Val(Sgnl)"=w3844) -> ()  [unwired: 2 in, 2 out]
                                }
                                }
                                }
                                }
                                }
                                }
                                }
                                }
                                }
                                frame "Image" {
                                n2551 = property on="Confocal Image" class="Bool (strict)"("Val(Sgnl)"=TRUE ("Value (Signaling)")) -> ()  [unwired: 2 in, 2 out]
                                }
                              }
                              n2552 = local write "Fl. High"(FALSE ("Fl. High")) -> ()
                              n2553 = local read "Time (s)"() -> (w3780:dbl)
                            }
                            frame #1 {
                              n2554 = case shown="True" "Auto F Reset" {
                                tunnel: w3852 -> [_ w3857]
                                tunnel: w3851 -> [_ w3856]
                                tunnel: w3850 -> [_ w3855]
                                tunnel: w3849 -> [_ w3854]
                                frame False {
                                }
                                frame True {
                                n2555 = node-c288() -> (w3859:T37)  [unwired: 4 in]
                                n2556 = timed-loop {
                                timing: w3859 -> [_]
                                timing-out: [_] -> w3858
                                tunnel: w3857 -> [w3864]
                                tunnel: w3856 -> [w3863]
                                tunnel: w3855 -> [w3862]
                                tunnel: w3854 -> [w3861]
                                stop <- w3860 stop-if-true
                                n2557 = node-c288() -> ()  [unwired: 1 in, 1 out]
                                n2558 = local read "Fl. Delta Thresh. (kHz)"() -> (w3873:dbl)
                                n2559 = local read "APD to Watch"() -> (w3874:bool)
                                n2560 = local read "Delta Fl. 1"() -> (w3875:dbl)
                                n2561 = local read "Delta Fl. 2"() -> (w3876:dbl)
                                n2562 = local read "Fl. Triggered..."() -> (w3867:bool)
                                n2563 = local read "Stop All"() -> (w3868:bool)
                                n2564 = local read "Reset Force"() -> (w3866:bool)
                                n2565 = Multiply(x=w3873, y=1000.0) -> (x*y=w3871:dbl)
                                n2566 = Select(t=w3875, s=w3874, f=w3876) -> (s? t:f=w3870:dbl)
                                n2567 = Not(x=w3867) -> (.not. x?=w3865:bool)
                                n2568 = Greater?(x=w3870, y=w3871) -> (0:w3869:bool)
                                n2569 = Compound Arithmetic op=OR(w3869, w3868, w3865, w3866) -> (w3860:bool)
                                n2570 = case shown="True" w3860 {
                                tunnel: w3864 -> [_ w3880]
                                tunnel: w3863 -> [_ w3884]
                                tunnel: w3862 -> [_ w3883]
                                tunnel: w3861 -> [_ w3882]
                                frame False {
                                }
                                frame True {
                                n2571 = case shown="\"Yank\"" w3884 {
                                tunnel: w3883 -> [_ w3894]
                                tunnel: w3882 -> [_ w3892]
                                frame "Image", Default {
                                }
                                frame "Yank" {
                                n2572 = flat-sequence {
                                tunnel: [w3897] -> w3895
                                tunnel: w3894 -> [w3897]
                                tunnel: [w3896] -> w3893
                                tunnel: w3892 -> [w3896]
                                tunnel: w3895 -> [w3903]
                                tunnel: w3893 -> [w3901]
                                frame #0 {
                                n2573 = local read "Yank Delay (s)"() -> (w3900:dbl)
                                n2574 = Multiply(x=w3900, y=1000.0) -> (x*y=w3898:dbl)
                                n2575 = Wait (ms)(milliseconds to wait=w3898) -> ()  [unwired: 1 out]
                                }
                                frame #1 {
                                n2576 = local read "Yank to which?"() -> (w3902:bool)
                                n2577 = case shown="False" w3902 {
                                tunnel: w3903 -> [_ w3931]
                                tunnel: w3901 -> [w3904 _]
                                frame False {
                                n2578 = flat-sequence {
                                tunnel: w3904 -> [w3905]
                                frame #0 {
                                n2579 = property on="Trap Pos FB SP" class="DigNum (strict)"("Val(Sgnl)"=w3905) -> ()  [unwired: 2 in, 2 out]
                                }
                                frame #1 {
                                n2580 = Wait (ms)(milliseconds to wait=u32 700) -> ()  [unwired: 1 out]
                                }
                                frame #2 {
                                n2581 = local read "Action (%)"() -> (w3910:dbl)
                                n2582 = Absolute Value(x=w3910) -> (abs(x)=w3909:dbl)
                                n2583 = Greater?(x=w3909, y=70.0) -> (0:w3907:bool)
                                n2584 = property on="Remove Action Offset" class="Bool (strict)"("Val(Sgnl)"=w3907) -> ()  [unwired: 2 in, 2 out]
